vi "Ignition Main.vi"(8 "error in":errorcluster, 9 "URL":string, 10 "folder name":string="NonUDT", 11 "Sequence Context In":refnum<k7>) -> (0 "error out":errorcluster)   [LabVIEW 2019, in "Ignition.lvlib"]
uses:
  Ignition.lvlib
  Tester Tx.ctl
  <vilib>/OPCUA/NI OPC UA Client.lvlib
panel:
  out "Tester Tx":T1
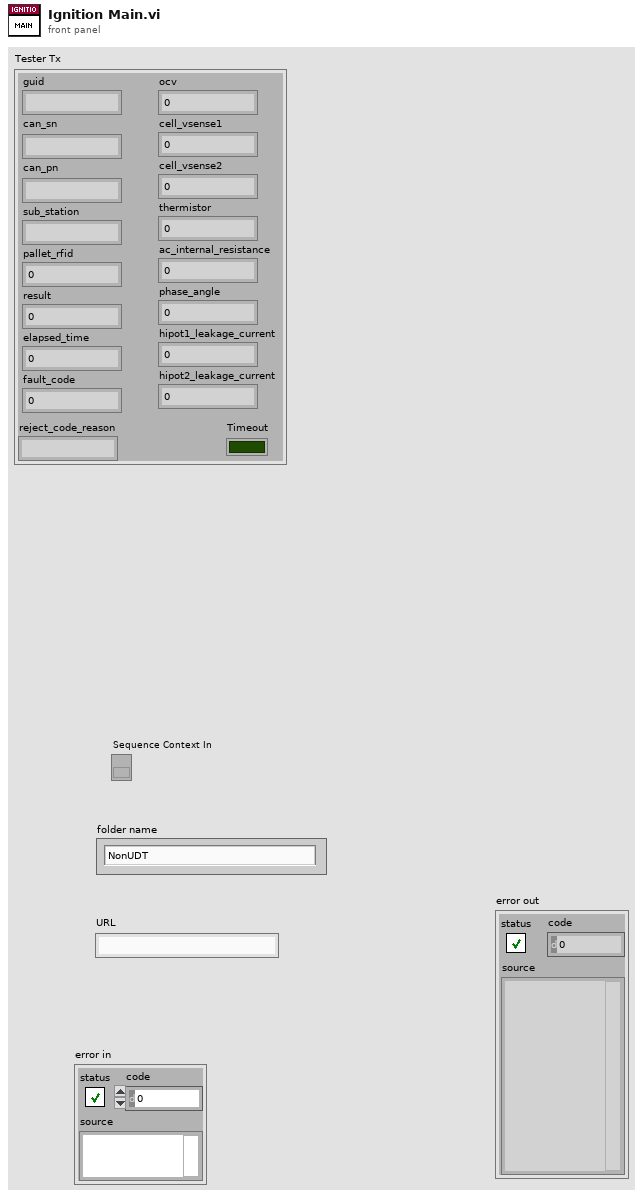
[diagram p1: front panel]
types:
  T1 = typedef "Ignition.lvlib/Tester Tx.ctl" = cluster{"thermistor":dbl, "phase_angle":dbl, "pallet_rfid":dbl, "ocv":dbl, "cell_vsense1":dbl, "cell_vsense2":dbl, "hipot1_leakage_current":dbl, "hipot2_leakage_current":dbl, "guid":string, "can_sn":string, "can_pn":string, "ac_internal_resistance":dbl, "sub_station":string, "fault_code":i32, "elapsed_time":i32, "result":i32, "reject_code_reason":string, "Timeout":bool}
  T2 = typedef "OPC UA Client Refnum.ctl" = refnum<k21>
  T3 = typedef "Subscription ID.ctl" = u32
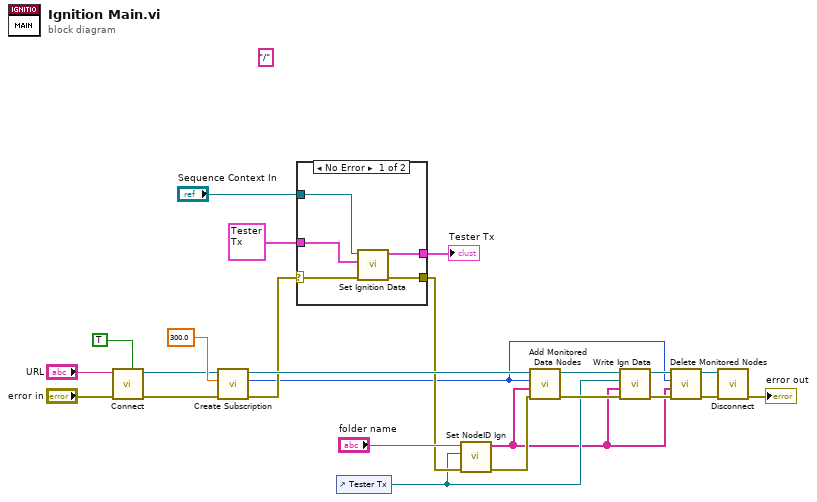
[diagram p0: block diagram]
diagram:
  (unwired) "/" ("Deliminated Char")
  n1 = call <vilib>:"Connect.vi"("trust any server (F)"=TRUE, "error in (no error)"="error in", "server endpoint URL"="URL") -> ("error out"=w23:errorcluster, "OPC UA client refnum out"=w22:T2)  [unwired: 6 in, 1 out]
  n2 = call <vilib>:"Create Subscription.vi"("error in (no error)"=w23, "publishing interval (1000 ms)"=300.0, "OPC UA client refnum in"=w22) -> ("error out"=w13:errorcluster, "subscription ID out"=w1:T3, "OPC UA client refnum out"=w19:T2)  [unwired: 4 in, 2 out]
  n3 = case shown="No Error" w13 {
    selector: w13 -> [w28 w30]
    tunnel: T1 {"thermistor"=0.0, "phase_angle"=0.0, "pallet_rfid"=0.0, "ocv"=0.0, "cell_vsense1"=0.0, "cell_vsense2"=0.0, "hipot1_leakage_current"=0.0, "hipot2_leakage_current"=0.0, "guid"="", "can_sn"="", "can_pn"="", "ac_internal_resistance"=0.0, "sub_station"="", "fault_code"=0, "elapsed_time"=0, "result"=0, "reject_code_reason"="", "Timeout"=FALSE} ("Tester Tx") -> [w29 w31]
    tunnel: "Sequence Context In" -> [w27 _]
    tunnel: [w26 w31] -> w14
    tunnel: [w25 w30] -> w12
    frame No Error {
      n4 = call "Set Ignition Data.vi"("error in"=w28, "Tester Tx"=w29, "Sequence Context"=w27) -> ("error out"=w25:errorcluster, "Tester Tx out"=w26:T1)  [unwired: 7 in]
    }
    frame Error {
    }
  }
  "Tester Tx" <- w14
  n5 = control-ref of="Tester Tx"() -> (w8:refnum<vi>)
  n6 = call "Set NodeID Ign.vi"("error in (no error)"=w12, "Control ref"=w8, "folder name"="folder name") -> ("error out"=w11:errorcluster, "NodeIDs"=w3:string[])  [unwired: 7 in]
  n7 = call <vilib>:"Add Monitored Data Nodes.vi"("error in (no error)"=w11, "node IDs"=w3, "subscription ID in"=w1, "OPC UA client refnum in"=w19) -> ("error out"=w10:errorcluster, "OPC UA client refnum out"=w9:T2)  [unwired: 4 in, 2 out]
  n8 = call "Write Ign Data.vi"("error in (no error)"=w10, "NodeIDs"=w3, "Control Ref"=w8, "OPC UA client refnum"=w9) -> ("error out"=w5:errorcluster, "OPC UA client refnum"=w6:T2)  [unwired: 6 in]
  n9 = call <vilib>:"Delete Monitored Nodes.vi"("error in (no error)"=w5, "node IDs"=w3, "subscription ID in"=w1, "OPC UA client refnum in"=w6) -> ("error out"=w4:errorcluster, "OPC UA client refnum out"=w2:T2)  [unwired: 3 in, 3 out]
  n10 = call <vilib>:"Disconnect.vi"("error in (no error)"=w4, "OPC UA client refnum in"=w2) -> ("error out"=→"error out":errorcluster)  [unwired: 9 in]
